vi "test tag value mode.vi"() -> ()   [LabVIEW 2017]
uses:
  13bbe123-394d-4020-95ca-253ea5abddb0.vi
  API-String-Arugments-Support/_Support/Convert API String Arguments to Data(variant).vi
panel:
  out "string 2":string
  in  "string":string
  out "error":errorcluster
  out "Data":errorcluster
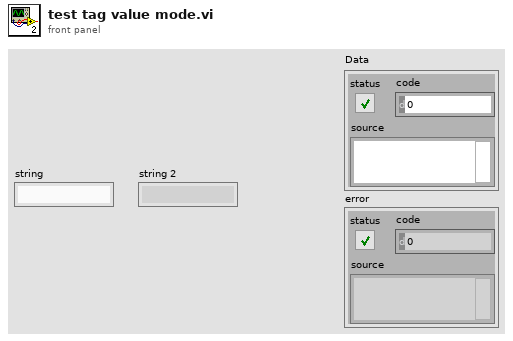
[diagram p1: front panel]
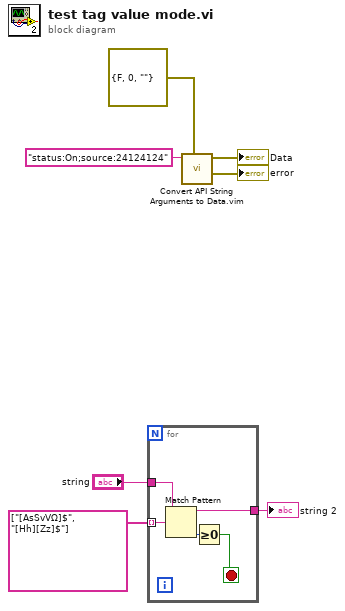
[diagram p0: block diagram]
diagram:
  n1 = for {
    tunnel: string[] ["[AsSvVΩ]$", "[Hh][Zz]$"] ("regular expression") -> [w12] mode=indexing
    tunnel: "string" -> [w11]
    tunnel: [w10] -> w1
    stop <- w8 stop-if-true
    n2 = Match Pattern(string=w11, regular expression=w12) -> (before substring=w10:string, offset past match=w9:i32)  [unwired: 1 in, 2 out]
    n3 = Greater Or Equal To 0?(x=w9) -> (x >= 0?=w8:bool)
  }
  "string 2" <- w1
  n4 = call "Convert API String Arguments to Data.vim"("Type"=errorcluster {"status"=FALSE, "code"=0, "source"=""} ("error in (no error)"), "String"="status:On;source:24124124") -> ("error"=→"error":errorcluster, "Data"=→"Data":errorcluster)  [unwired: 6 in]
